vi "S7_Error_Reconnect_TCP.vi"(8 "error in":errorcluster, 9 "Timeout":u32=5000, 10 "IP Address":string, 11 "TCP Connection Ref":refnum<k5>) -> (0 "error out":errorcluster, 3 "TCP Connection Ref Out":refnum<k5>)   [LabVIEW 2017, in "S7 TCP.lvlib"]
uses:
  S7 TCP.lvlib
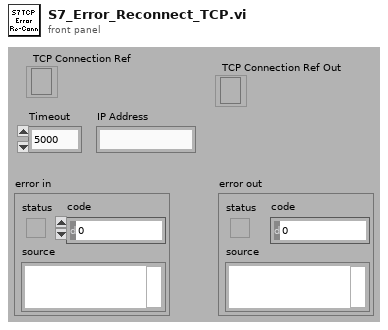
[diagram p1: front panel]
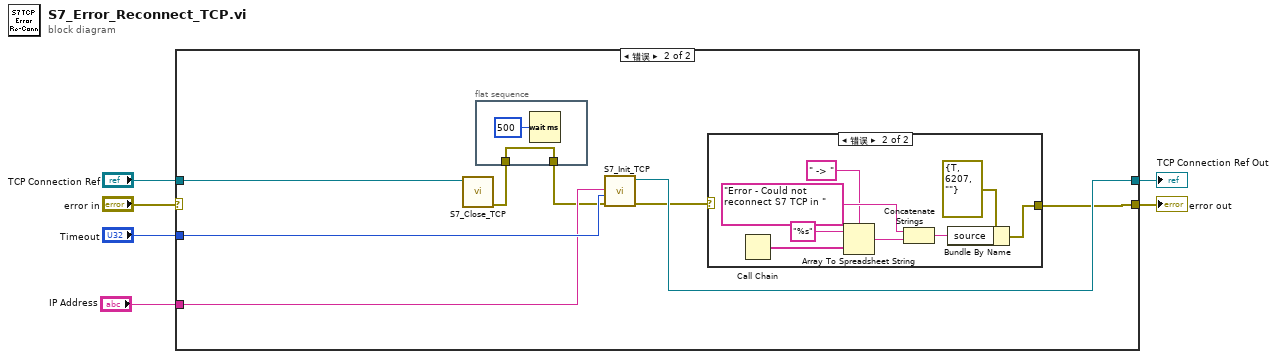
[diagram p0: block diagram]
diagram:
  n1 = case shown="错误" "error in" {
    selector: "error in" -> [w7 _]
    tunnel: [w8 w14] -> w3
    tunnel: [w7 w13] -> w5
    tunnel: "TCP Connection Ref" -> [w8 w16]
    tunnel: "Timeout" -> [_ w15]
    tunnel: "IP Address" -> [_ w12]
    frame No Error {
    }
    frame Error {
      n2 = call "S7_Close_TCP.vi"("TCP Connection Ref"=w16) -> ("error out"=w10:errorcluster)  [unwired: 2 in, 8 out]
      n3 = flat-sequence {
        tunnel: w10 -> [w17]
        tunnel: [w17] -> w9
        frame #0 {
          n4 = Wait (ms)(milliseconds to wait=u32 500) -> ()  [unwired: 1 out]
        }
      }
      n5 = call "S7_Init_TCP.vi"("error in"=w9, "Connection Timeout"=w15, "IP Address"=w12) -> ("error out"=w11:errorcluster, "TCP Connection Ref"=w14:refnum<k5>)  [unwired: 2 in, 5 out]
      n6 = case shown="错误" w11 {
        selector: w11 -> [w19 _]
        tunnel: [w19 w20] -> w13
        frame No Error {
        }
        frame Error {
          n7 = Call Chain() -> (call chain=w24:string[])
          n8 = Array To Spreadsheet String(delimiter (Tab)=" -> ", array=w24, 3:"%s" ("format string")) -> (spreadsheet string=w23:string)
          n9 = Concatenate Strings("Error - Could not reconnect S7 TCP in " ("source"), w23) -> (w25:string)
          n10 = Bundle By Name(cluster=errorcluster {"status"=TRUE, "code"=6207, "source"=""} ("error out"), "source"=w25) -> (w20:errorcluster)
        }
      }
    }
  }
  "error out" <- w5
  "TCP Connection Ref Out" <- w3
